vi "main.vi"() -> ()   [LabVIEW 2011]
uses:
  vehicleCluster.ctl
panel:
  out "VehicleCluster 2":T1={"NumberOfWheels"=0.0, "Name"="sdf"}
  out "nameOut":string
  in  "VehicleCluster":T1
  out "numberOfWheelsOut":dbl
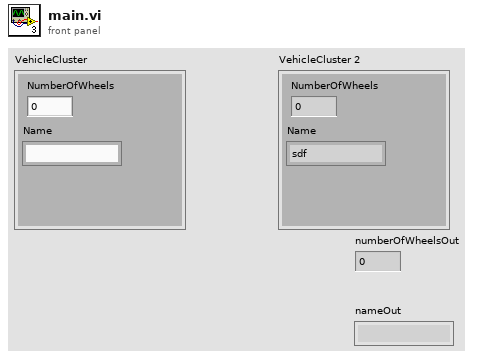
[diagram p1: front panel]
types:
  T1 = typedef "vehicleCluster.ctl" = cluster{"NumberOfWheels":dbl, "Name":string}
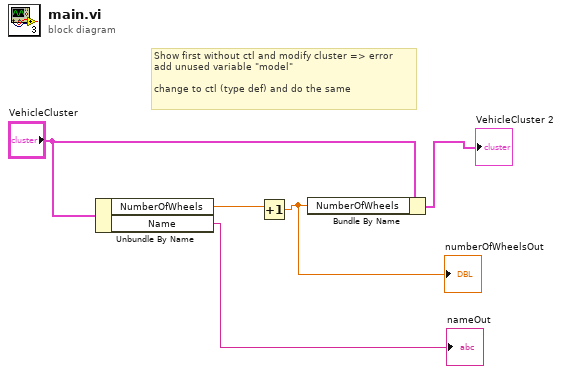
[diagram p0: block diagram]
diagram:
  # "Show first without ctl and modify cluster => error\nadd unused variable \"model\"\n\nchange to ctl (type def) and do the same"
  n1 = Unbundle By Name("VehicleCluster") -> ("NumberOfWheels"=w5:dbl, "Name"=→"nameOut":string)
  n2 = Increment(x=w5) -> (x+1=w3:dbl)
  "numberOfWheelsOut" <- w3
  n3 = Bundle By Name(cluster="VehicleCluster", "NumberOfWheels"=w3) -> (→"VehicleCluster 2":T1)
